vi "Task from tool.vi"(8 "Too large":dbl=12.0 format="%#_13g", 9 "Object lengh":dbl, 10 "Tool":dbl, 11 "Assignment - Task":string) -> (2 "Task to String":string, 3 "Assignment":string)   [LabVIEW 2024]
doc: "Assigning robot task, given the previesly selected tool."
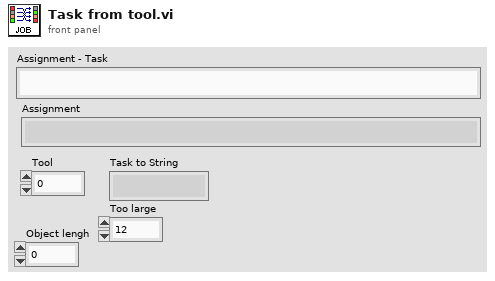
[diagram p1: front panel]
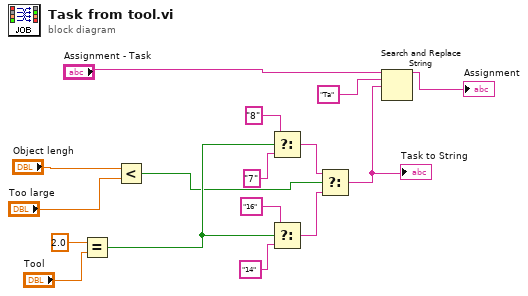
[diagram p0: block diagram]
diagram:
  n1 = Equal?(x=2.0, y="Tool") -> (x = y?=w7:bool)
  n2 = Less?(x="Object lengh", y="Too large") -> (x < y?=w2:bool)
  n3 = Select(t="8", s=w7, f="7") -> (s? t:f=w6:string)
  n4 = Select(t="16", s=w7, f="14") -> (s? t:f=w5:string)
  n5 = Select(t=w6, s=w2, f=w5) -> (s? t:f=w4:string)
  "Task to String" <- w4
  n6 = Search and Replace String(input string="Assignment - Task", search string="Ta", replace string=w4) -> (result string=→"Assignment":string)  [unwired: 5 in, 3 out]
